vi "DelayRight.vi"(2 "sample in":fxp<+/-,25,16>, 3 "n":u32) -> (0 "SampleOut":fxp<+/-,25,16>)   [LabVIEW 2016]
uses:
  Global 1.vi
  <vilib>/rvi/DataTransferAndStorage/Container/XNode/niFpgaContainer.xnode
  <vilib>/rvi/Memory/Memory_Emulation/nirvimemoryEmulation.vi
  <vilib>/rvi/Memory/Memory_Emulation/nirvimemoryFastEmulation.vi
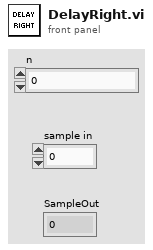
[diagram p1: front panel]
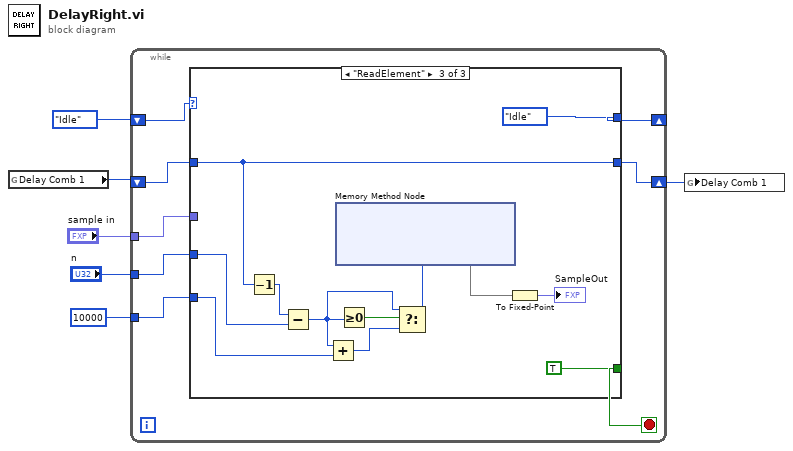
[diagram p0: block diagram]
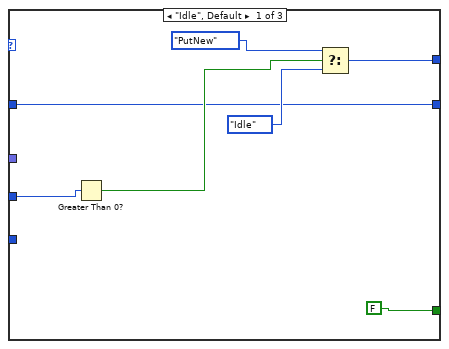
[diagram p2: hidden frame]
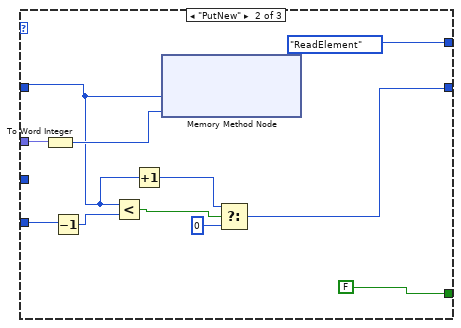
[diagram p3: hidden frame]
diagram:
  n1 = global read "Global 1.vi" "Delay Comb 1"() -> (w5:u32)
  n2 = while {
    shift-right: [w12] -> _
    shift-left: enum16{"Idle", "PutNew", "ReadElement"}."Idle" -> [w14]
    shift-right: [w11] -> w3
    shift-left: w5 -> [w10]
    tunnel: "n" -> [w13]
    tunnel: "sample in" -> [w9]
    tunnel: u32 10000 -> [w8]
    stop <- w7 stop-if-true
    n3 = case shown="\"ReadElement\"" w14 {
      tunnel: w13 -> [w21 _ w42]
      tunnel: [w17 enum16{"Idle", "PutNew", "ReadElement"}."ReadElement" enum16{"Idle", "PutNew", "ReadElement"}."Idle"] -> w12
      tunnel: [w16 w27 w41] -> w11
      tunnel: w10 -> [w16 w22 w41]
      tunnel: w9 -> [_ w24 _]
      tunnel: w8 -> [_ w32 w40]
      tunnel: [FALSE FALSE TRUE] -> w7
      frame "Idle", Default {
        n4 = Greater Than 0?(x=w21) -> (x > 0?=w20:bool)
        n5 = Select(t=enum16{"Idle", "PutNew", "ReadElement"}."PutNew", s=w20, f=enum16{"Idle", "PutNew", "ReadElement"}."Idle") -> (s? t:f=w17:enum16{"Idle", "PutNew", "ReadElement"})
      }
      frame "PutNew" {
        n6 = To Word Integer(number=w24) -> (16bit integer=w23:i16)
        n7 = Decrement(x=w32) -> (x-1=w31:u32)
        n8 = Less?(x=w22, y=w31) -> (x < y?=w29:bool)
        n9 = Increment(x=w22) -> (x+1=w30:u32)
        n10 = xnode ("Memory Method Node")("Address"=w22, "Data"=w23) -> ()  [unwired: 1 in, 1 out]
        n11 = Select(t=w30, s=w29, f=u32 0) -> (s? t:f=w27:u32)
      }
      frame "ReadElement" {
        n12 = Decrement(x=w41) -> (x-1=w43:u32)
        n13 = Subtract(x=w43, y=w42) -> (x-y=w37:u32)
        n14 = Add(x=w37, y=w40) -> (x+y=w38:u32)
        n15 = Greater Or Equal To 0?(x=w37) -> (x >= 0?=w39:bool)
        n16 = Select(t=w37, s=w39, f=w38) -> (s? t:f=w33:u32)
        n17 = xnode ("Memory Method Node")("Address"=w33) -> ("Data"=w34)  [unwired: 1 in, 1 out]
        n18 = To Fixed-Point(number=w34) -> (fixed-point=→"SampleOut":fxp<+/-,25,16>)  [unwired: 1 in]
      }
    }
  }
  n19 = global write "Global 1.vi" "Delay Comb 1"(w3) -> ()
